vi "Configure Math Expression.vi"   [LabVIEW 2011, in "Tektronix 7000 Series.lvlib"]
doc: "This polymorphic VI creates mathematical expressions with different numbers of operands.\n\nThe Configure Math Expression (Unary) VI creates a mathematical expression with one operand.\n\nThe Configure Math Expression (Binary) VI creates a mathematical expression with two operands."
uses:
  Tektronix 7000 Series.lvlib
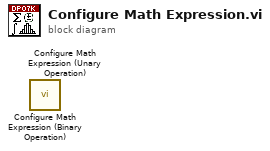
[diagram p0: block diagram]
diagram:
  n1 = call "Configure Math Expression (Binary Operation).vi"() -> ()  [unwired: 9 in, 3 out]
  n2 = call "Configure Math Expression (Unary Operation).vi"() -> ()  [unwired: 9 in, 3 out]
